vi "Log State.vi"(8 "error in":errorcluster, 10 "Model Status":T3, 11 "Data":T1) -> (0 "error out":errorcluster, 3 "Data out":T1)   [LabVIEW 2014, in "Logger.lvlib"]
uses:
  Logger.lvlib
  Model/TypeDefs/Get Model Status Control.ctl
  Model/Model.lvlib
  TypeDefs/Logger State.ctl
  TypeDefs/Logger Data.ctl
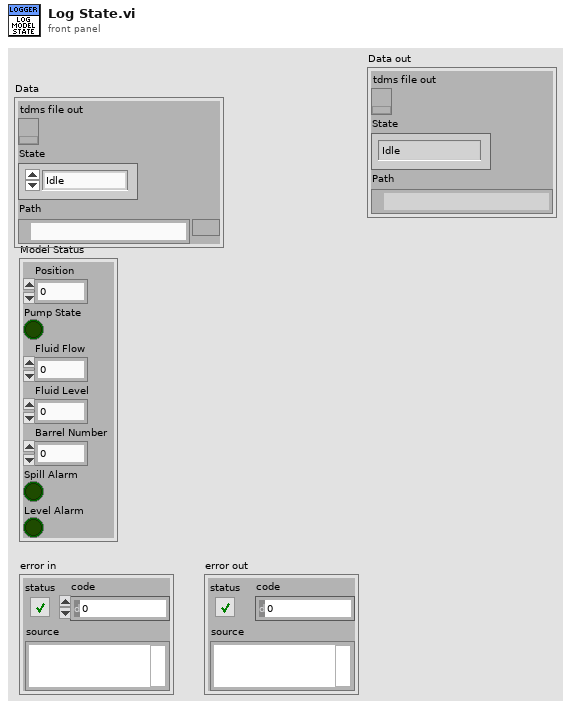
[diagram p1: front panel]
types:
  T1 = typedef "Logger.lvlib/Logger Data.ctl" = cluster{"tdms file out":refnum<k34>, "State":T2, "Path":path}
  T2 = typedef "Logger.lvlib/Logger State.ctl" = enum16{"Idle", "Working"}
  T3 = typedef "Model.lvlib/Get Model Status Control.ctl" = cluster{"Position":dbl, "Pump State":bool, "Fluid Flow":dbl, "Fluid Level":dbl, "Barrel Number":i32, "Spill Alarm":bool, "Level Alarm":bool}
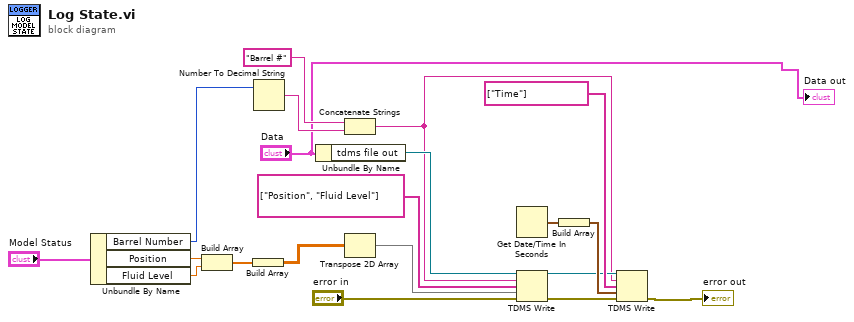
[diagram p0: block diagram]
diagram:
  n1 = Unbundle By Name("Model Status") -> ("Barrel Number"=w6:i32, "Position"=w11:dbl, "Fluid Level"=w12:dbl)
  n2 = Build Array(w11, w12) -> (w18:dbl[])
  n3 = Build Array(w18) -> (w19:dbl[][])
  n4 = Number To Decimal String(number=w6) -> (decimal integer string=w4:string)  [unwired: 1 in]
  n5 = Unbundle By Name("Data") -> ("tdms file out"=w9:refnum<k34>)
  n6 = Concatenate Strings("Barrel #", w4) -> (w3:string)
  n7 = Transpose 2D Array(2D array=w19) -> (transposed array=w20:dbl[][])
  n8 = Get Date/Time In Seconds() -> (seconds since 1Jan1904=w16:timestamp)
  n9 = TDMS Write(0:w9, 5:w3, 7:string[] ["Position", "Fluid Level"], 9:w20, 11:"error in") -> (4:w14:refnum<k34>, 15:w13:errorcluster)  [unwired: 1 in, 2 out]
  n10 = Build Array(w16) -> (w17:timestamp[])
  n11 = TDMS Write(0:w14, 5:w3, 7:string[] ["Time"], 9:w17, 11:w13) -> (15:→"error out":errorcluster)  [unwired: 1 in, 3 out]
  "Data out" <- "Data"
